vi "Write hkParam.vi"(8 "error in (no error)":errorcluster, 10 "hkParam":T1={"rhDilFac"=1.0, "Q"=0.0, "Tmean"=0.0, "extDilFac"=1.0, "rhCell"=0.0, "P"=0.0, "T"=0.0}, 11 "CRDS Cell Data in":refnum<class "CRDS Cell Data.lvclass">) -> (0 "error out":errorcluster, 3 "CRDS Cell Data out":refnum<class "CRDS Cell Data.lvclass">)   [LabVIEW 2015, in "CRDS Lib.lvlib" / "CRDS Cell Data.lvclass"]
uses:
  CRDS Cell Data.lvclass
  Cell/hkParam Ctl.ctl
  CRDS Cell Data.lvclass/CRDS Cell Data.ctl
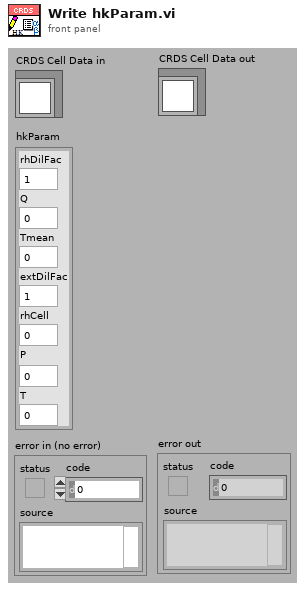
[diagram p1: front panel]
types:
  T1 = typedef "CRDS Lib.lvlib/CRDS Cell Data.lvclass/hkParam Ctl.ctl" = cluster{"rhDilFac":sgl, "Q":sgl, "Tmean":sgl, "extDilFac":sgl, "rhCell":sgl, "P":sgl, "T":sgl}
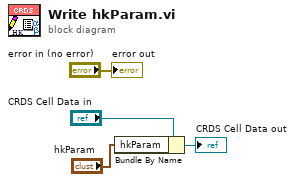
[diagram p0: block diagram]
diagram:
  n1 = Bundle By Name(cluster="CRDS Cell Data in", "hkParam"="hkParam") -> (→"CRDS Cell Data out":refnum<class "CRDS Cell Data.lvclass">)
  "error out" <- "error in (no error)"
